vi "Z6_Beamline_Chief.publish Ready to Shot.vi"(0 "i ref in":refnum<vi>, 2 "R2S before":bool, 5 "error in (no error)":errorcluster) -> (14 "i ref out":refnum<vi>, 19 "error out":errorcluster)   [LabVIEW 2014, in "Z6_Beamline_Chief.lvlib"]
doc: "This VI sets whether the R2S-Information (\"ready to shot\") to own attributes, and publishes it as DIM service."
uses:
  Z6_Beamline_Chief.lvlib
  lib.lib/DimLVEvent/LVDimInterface/LVDimInterface.lvlib
  PH_BL-Master/PH_BL-Master.lvlib
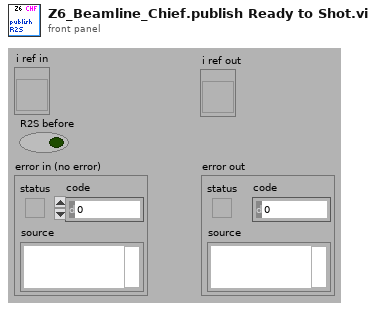
[diagram p1: front panel]
types:
  T1 = typedef "PH_BL-Master.lvlib/PH_BL-Master.i attribute.ctl" = cluster{"Remote controlled":bool, "Boolean Condition Service Subscriber":refnum<vi>[], "Picture Condition Service Subscriber":refnum<vi>[], "R2S":cluster{"GUI Ref":refnum<vi>, "State":bool}, "Vacua":cluster{"GUI Ref":refnum<vi>, "Limit":dbl, "Curr Value":dbl, "in range":bool}[], "O2 Inspection":cluster{"GUI Ref":refnum<vi>, "Concentration":dbl, "State":T2}[], "Boolean Status Service Subscriber":cluster{"GUI Ref":refnum<vi>, "Status":T2, "no Link?":bool, "Status Subscriber Class":T3}[], "Picture Status Service Subscriber":cluster{"GUI Ref":refnum<vi>, "Status":T2, "no Link?":bool, "Status Subscriber Class":T3}[], "6P 4Q Service Subscriber":cluster{"GUI Ref":refnum<vi>, "Selector":T4, "no Link?":bool}[], "Index of latest 6P 4Q changing Instance":i32, "Index of latest Picture Status changing Instance":i32, "Index of latest Boolean Status changing Instance":i32, "Vision ID on same Node":string, "Start Phase over?":bool, "GUI Ref Delete":refnum<vi>}
  T2 = typedef "PH_StatusHandler.lvlib/PH_StatusHandler.Status.ctl" = i16
  T3 = typedef "PH_BL-Master.lvlib/PH_BL-Master.Status Subscriber Class.ctl" = enum16{"unknown", "Switch", "BB", "6P Switch", "Switch GUI", "Switch and 6P State", "Force Sensor"}
  T4 = typedef "PH_4_Pos_Selector.lvlib/PH_4_Pos_Selector.Position Selector.ctl" = u16
  T5 = typedef "Z6_Beamline_Chief.lvlib/Z6_Beamline_Chief.i attribute.ctl" = cluster{"R2S Service ID":i32}
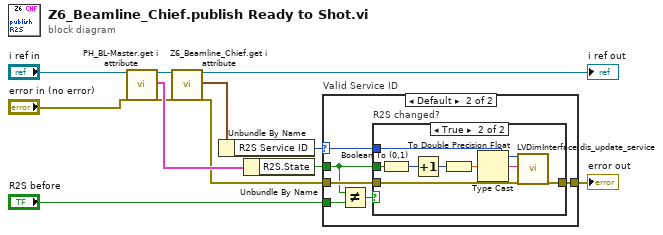
[diagram p0: block diagram]
diagram:
  n1 = call "PH_BL-Master.get i attribute.vi"("i ref in"="i ref in", "error in (no error)"="error in (no error)") -> ("i ref out"=w7:refnum<vi>, "i attribute"=w10:T1, "error out"=w6:errorcluster)  [unwired: 15 in]
  n2 = call "Z6_Beamline_Chief.get i attribute.vi"("i ref in"=w7, "error in (no error)"=w6) -> ("i ref out"=→"i ref out":refnum<vi>, "i attribute"=w4:T5, "error out"=w5:errorcluster)  [unwired: 15 in]
  n3 = Unbundle By Name(w4) -> ("R2S Service ID"=w3:i32)
  n4 = Unbundle By Name(w10) -> ("R2S.State"=w2:bool)
  n5 = case "Valid Service ID" shown="Default" w3 {
    selector: w3 -> [_ w17]
    tunnel: w5 -> [w13 w19]
    tunnel: [w13 w18] -> w11
    tunnel: w2 -> [_ w15]
    tunnel: "R2S before" -> [_ w16]
    frame -1 {
    }
    frame Default {
      n6 = Not Equal?(x=w15, y=w16) -> (x != y?=w14:bool)
      n7 = case "R2S changed?" shown="True" w14 {
        tunnel: w19 -> [w20 w27]
        tunnel: [w20 w26] -> w18
        tunnel: w17 -> [_ w22]
        tunnel: w15 -> [_ w21]
        frame False {
        }
        frame True {
          n8 = Boolean To (0,1)(Boolean=w21) -> (0, 1=w25:i16)
          n9 = Increment(x=w25) -> (x+1=w24:i16)
          n10 = To Double Precision Float(number=w24) -> (double precision float=w23:dbl)
          n11 = Type Cast(x=w23) -> (*(type *) &x=w28:string)  [unwired: 1 in]
          n12 = call "LVDimInterface.dis_update_service.vi"("my_serviceID"=w22, "data"=w28, "error in (no error)"=w27) -> ("error out"=w26:errorcluster)  [unwired: 14 in, 2 out]
        }
      }
    }
  }
  "error out" <- w11
